vi "Controller_Adrian_Debug.vi"(0 "name 2":string, 5 "port or service name":u16=16389, 7 "connection ID":refnum<k16>, 9 "error in (no error)":errorcluster, 11 "x":dbl[](array[numeric])) -> (4 "*(type *) &x":dbl[](array[numeric]), 6 "error out":errorcluster, 8 "connection ID out":refnum<k16>)   [LabVIEW 2021]
panel:
  in  "Stop":bool
  out "port":u16
  out "name":string
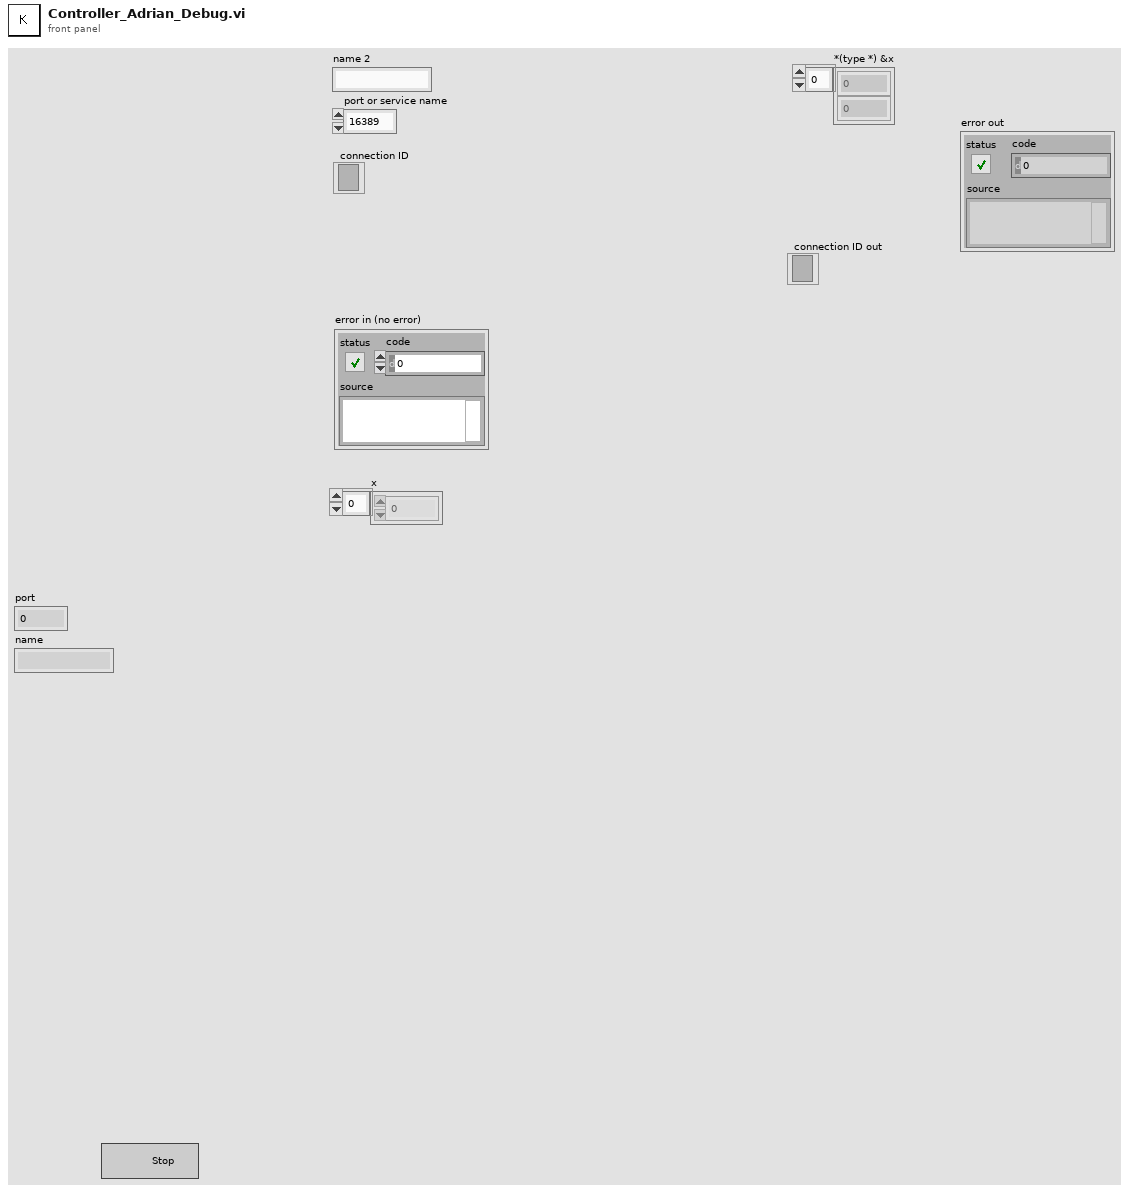
[diagram p1: front panel]
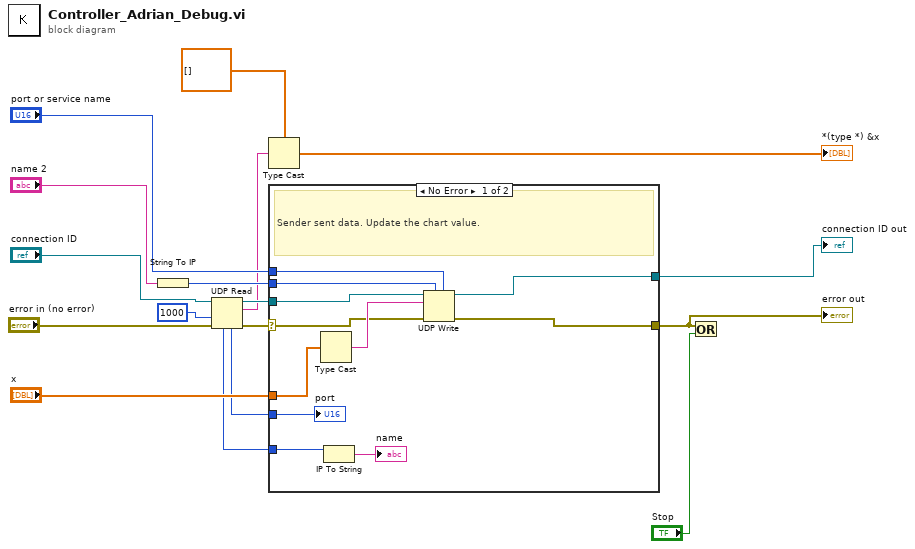
[diagram p0: block diagram]
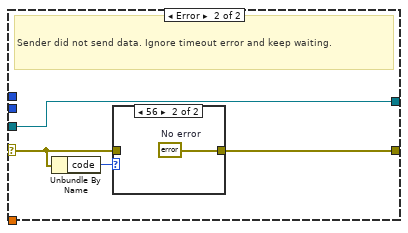
[diagram p2: hidden frame]
diagram:
  n1 = String To IP(1:"name 2") -> (0:w3:u32)
  n2 = UDP Read(connection ID="connection ID", timeout ms (25000)=1000, 8:"error in (no error)") -> (data out=w1:string, error out=w7:errorcluster, 3:w4:refnum<k16>, 4:w6:u16, 6:w5:u32)  [unwired: 1 out]
  n3 = Type Cast(type=dbl[] [], x=w1) -> (*(type *) &x=→"*(type *) &x":dbl[])
  n4 = case shown="No Error" w7 {
    selector: w7 -> [w19 w31]
    tunnel: [w18 w29] -> w12
    tunnel: [w28 w30] -> w11
    tunnel: w6 -> [w26 _]
    tunnel: w5 -> [w25 _]
    tunnel: w4 -> [w24 w30]
    tunnel: "port or service name" -> [w23 _]
    tunnel: w3 -> [w22 _]
    tunnel: "x" -> [w20 _]
    frame No Error {
      # "Sender sent data. Update the chart value."
      n5 = Type Cast(x=w20) -> (*(type *) &x=w21:string)  [unwired: 1 in]
      n6 = IP To String(2:w25) -> (0:→"name":string)  [unwired: 1 in]
      n7 = UDP Write(address=w22, port or service name=w23, connection ID=w24, data in=w21, 8:w19) -> (error out=w18:errorcluster, 3:w28:refnum<k16>)  [unwired: 1 in]
      "port" <- w26
    }
    frame Error {
      # "Sender did not send data. Ignore timeout error and keep waiting."
      n8 = Unbundle By Name(w31) -> ("code"=w32:i32)
      n9 = case shown="56" w32 {
        tunnel: w31 -> [w33 _]
        tunnel: [w33 w34] -> w29
        frame Default {
        }
        frame 56 {
          w34 = errorcluster {"status"=FALSE, "code"=0, "source"=""}  # No error
        }
      }
    }
  }
  "error out" <- w12
  "connection ID out" <- w11
  n10 = Or(x=w12, y="Stop") -> ()  [unwired: 1 out]
